vi "Start Widget Engine.vi"(8 "Error In":errorcluster) -> (0 "Error Out":errorcluster)   [LabVIEW 2013, in "Template.lvlib"]
uses:
  Template.lvlib
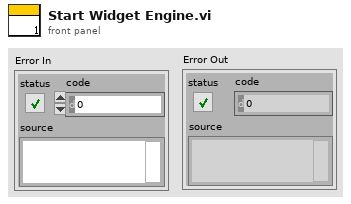
[diagram p1: front panel]
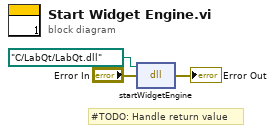
[diagram p0: block diagram]
diagram:
  # "#TODO: Handle return value"
  n1 = dll-call lib="?" fn="startWidgetEngine"(path in=path "C:/LabQt/LabQt.dll", error in="Error In") -> (error out=→"Error Out":errorcluster)  [unwired: 2 in, 1 out]
